vi "BlkReadFrame2.vi"(9 "BlkFilePath":path=path "D:/Expt/test/test1/test_red.blk") -> ()   [LabVIEW 2011]
panel:
  out "frameIndex":i64
  in  "等待时间（毫秒）":u32
  out "Image":T1(plugin-control)
  in  "skipFrame":i64
  out "datatype 2":u16(ring)=13 items=["U8"=11, "I16"=12, "U32"=13, "SGL"=14]
  out "SequenceOfID":u8[](array[numeric])
  out "Stimuli":i32
  out "FramesPerStim":i32
  out "FrameHeight":i32
  out "FrameWidth":i32
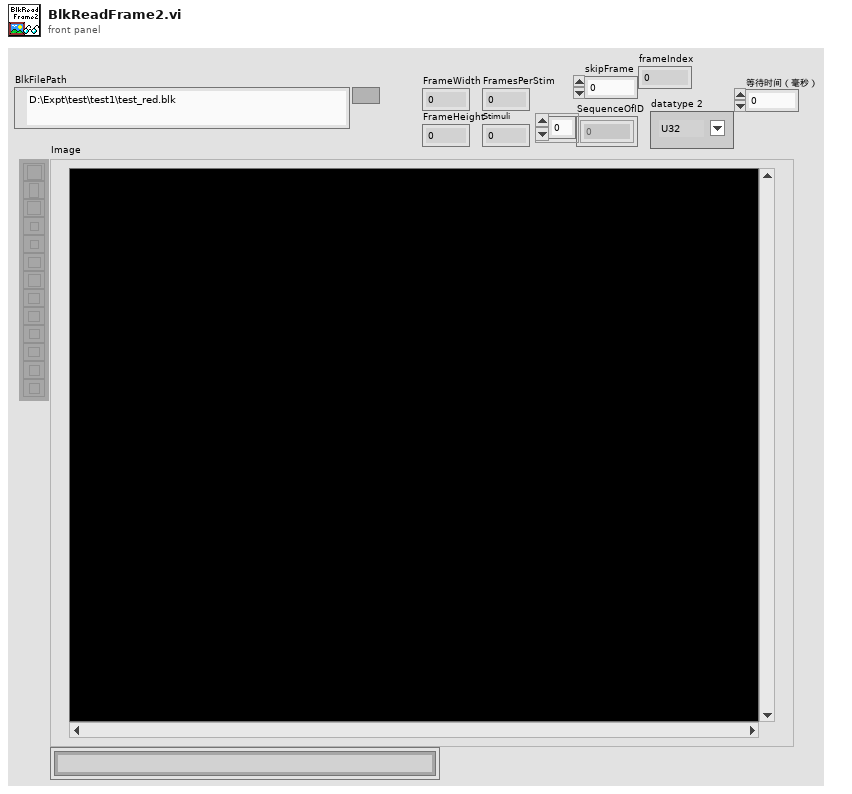
[diagram p1: front panel]
types:
  T1 = typedef "IMAQ Image.ctl" = refnum<image>
  T2 = typedef "Image Type" = u32
  T3 = enum16{"big-endian, network order", "native, host order", "little-endian"}
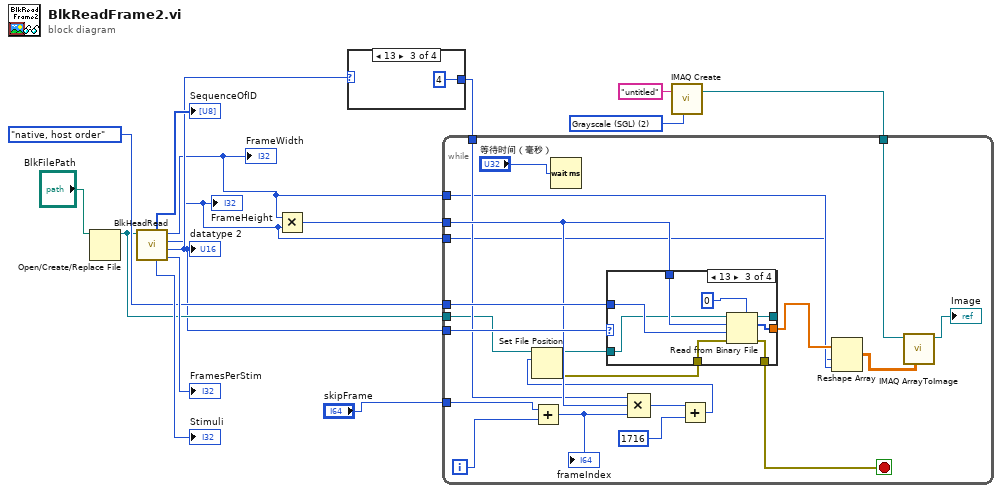
[diagram p0: block diagram]
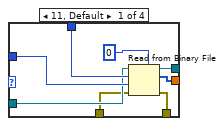
[diagram p2: hidden frame]
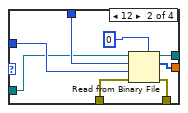
[diagram p3: hidden frame]
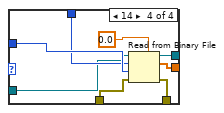
[diagram p4: hidden frame]
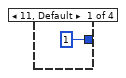
[diagram p5: hidden frame]
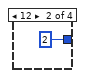
[diagram p6: hidden frame]
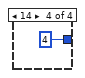
[diagram p7: hidden frame]
diagram:
  w2 = T2 2 items=["Grayscale (U8)", "Grayscale (I16)", "Grayscale (SGL)", "Complex (CSG)", "RGB (U32)", "HSL (U32)", "RGB (U64)", "Grayscale (U16)"] ("Image Type")
  n1 = Open/Create/Replace File(file path (use dialog)="BlkFilePath") -> (refnum out=w10:refnum<file>)  [unwired: 5 in, 2 out]
  n2 = call "BlkHeadRead.vi"("引用句柄"=w10) -> ("FramesPerStim"=→"FramesPerStim":i32, "datatype"=w9:i32, "FrameHeight"=w4:i32, "FrameWidth"=w5:i32, "Stimuli"=→"Stimuli":i32, "SequenceOfID"=→"SequenceOfID":u8[])  [unwired: 5 in]
  "FrameWidth" <- w5
  "FrameHeight" <- w4
  "datatype 2" <- w9
  n3 = Multiply(x=w5, y=w4) -> (x*y=w8:i32)
  n4 = case shown="13" w9 {
    tunnel: [i64 1 i64 2 i64 4 i64 4] -> w6
    frame 11, Default {
    }
    frame 12 {
    }
    frame 13 {
    }
    frame 14 {
    }
  }
  n5 = call "IMAQ Create"("Image Name"="untitled", "Image Type"=w2) -> ("New Image"=w1:T1)  [unwired: 3 in, 1 out]
  n6 = while {
    tunnel: T3."native, host order" ("字节顺序(0:big-endian, network order)") -> [w40]
    tunnel: w10 -> [w31]
    tunnel: w9 -> [w39]
    tunnel: w8 -> [w35]
    tunnel: "skipFrame" -> [w37]
    tunnel: w6 -> [w34]
    tunnel: w5 -> [w25]
    tunnel: w4 -> [w24]
    tunnel: w1 -> [w22]
    i -> [w38]
    stop <- w27 stop-if-true
    n7 = Add(x=w37, y=w38) -> (x+y=w36:i64)
    "frameIndex" <- w36
    n8 = Wait (ms)(milliseconds to wait="等待时间（毫秒）") -> ()  [unwired: 1 out]
    n9 = Compound Arithmetic op=MULTIPLY(w34, w35, w36) -> (w33:i64)
    n10 = Add(x=w33, y=i64 1716) -> (x+y=w30:i64)
    n11 = Set File Position(offset (in bytes) (0)=w30, refnum=w31) -> (refnum out=w29:refnum<file>, error out=w26:errorcluster)  [unwired: 2 in]
    n12 = case shown="13" w39 {
      tunnel: [w47 w55 w63 w71] -> w28
      tunnel: [w46 w54 w62 w70] -> _
      tunnel: w40 -> [w45 w53 w61 w69]
      tunnel: w35 -> [w44 w52 w60 w68]
      tunnel: w29 -> [w43 w51 w59 w67]
      tunnel: [w42 w50 w58 w66] -> w27
      tunnel: w26 -> [w41 w49 w57 w65]
      frame 11, Default {
        n13 = Read from Binary File(5:u8 0, 8:w41, 9:w45, 10:w44, 11:w43) -> (0:w42:errorcluster, 2:w47:u8[], 3:w46:refnum<file>)  [unwired: 1 in, 1 out]
      }
      frame 12 {
        n14 = Read from Binary File(5:u16 0, 8:w49, 9:w53, 10:w52, 11:w51) -> (0:w50:errorcluster, 2:w55:u16[], 3:w54:refnum<file>)  [unwired: 1 in, 1 out]
      }
      frame 13 {
        n15 = Read from Binary File(5:u32 0, 8:w57, 9:w61, 10:w60, 11:w59) -> (0:w58:errorcluster, 2:w63:u32[], 3:w62:refnum<file>)  [unwired: 1 in, 1 out]
      }
      frame 14 {
        n16 = Read from Binary File(5:sgl 0.0, 8:w65, 9:w69, 10:w68, 11:w67) -> (0:w66:errorcluster, 2:w71:sgl[], 3:w70:refnum<file>)  [unwired: 1 in, 1 out]
      }
    }
    n17 = Reshape Array(w28, w24, w25) -> (w23:sgl[][])
    n18 = call "IMAQ ArrayToImage"("Image Pixels (Float)"=w23, "Image"=w22) -> ("Image Out"=→"Image":T1)  [unwired: 8 in, 1 out]
  }
